vi "Toggle.vi"(1 "Trigger":bool) -> (0 "New_Mode":bool)   [LabVIEW 2018]
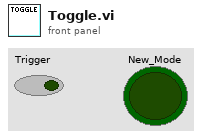
[diagram p1: front panel]
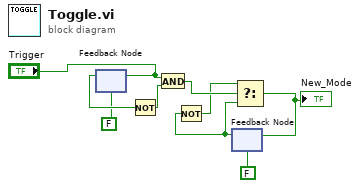
[diagram p0: block diagram]
diagram:
  n1 = feedback #1(FALSE ("Trigger")) -> (w8:bool)
  n2 = feedback-in #1("Trigger") -> ()
  n3 = Not(x=w8) -> (.not. x?=w6:bool)
  n4 = And(x="Trigger", y=w6) -> (x .and. y?=w5:bool)
  n5 = feedback #2(FALSE) -> (w3:bool)
  n6 = Not(x=w3) -> (.not. x?=w4:bool)
  n7 = Select(t=w4, s=w5, f=w3) -> (s? t:f=w2:bool)
  "New_Mode" <- w2
  n8 = feedback-in #2(w2) -> ()
